vi "Find Device by Multicolumn Listbox Value.vi"(3 "error in (no error)":errorcluster, 4 "Multicolumn Listbox":refnum<vi>, 5 "ACNET Devices":refnum<class "ACNET Devices.lvclass">) -> (0 "error out":errorcluster, 1 "Found?":bool, 2 "ACNET Device Cluster":T1)   [LabVIEW 2013, in "ACNET Monitor.lvlib"]
uses:
  ACNET Monitor.lvlib
  ACNET Devices.lvclass
  ACNET Device.lvclass
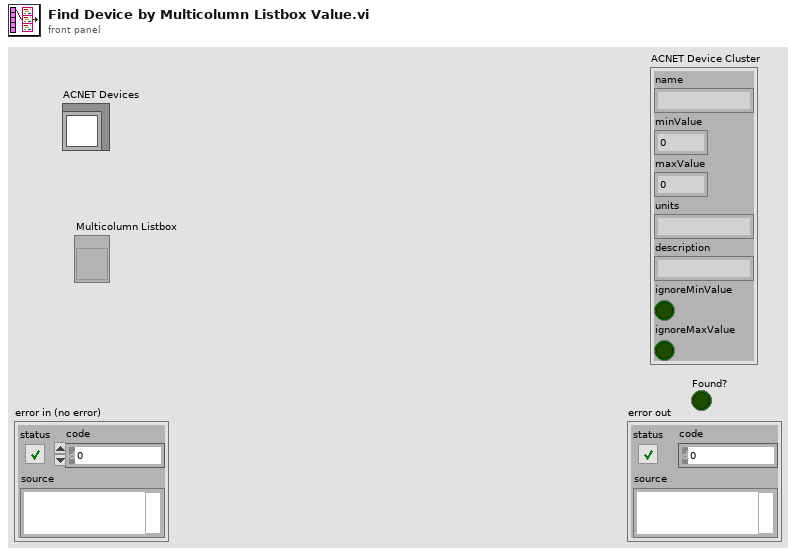
[diagram p1: front panel]
types:
  T1 = cluster{"name":string, "minValue":dbl, "maxValue":dbl, "units":string, "description":string, "ignoreMinValue":bool, "ignoreMaxValue":bool}
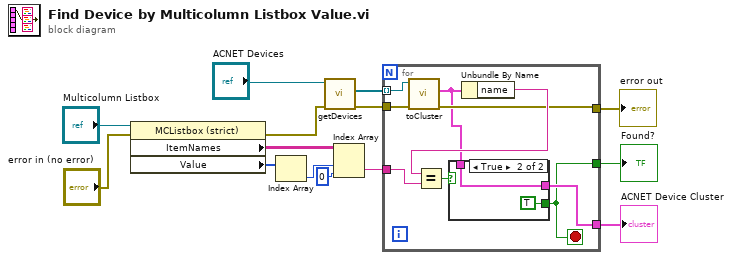
[diagram p0: block diagram]
diagram:
  n1 = property on="Property Node" class="MCListbox (strict)"(reference="Multicolumn Listbox", error in="error in (no error)") -> (error out=w10:errorcluster, "ItemNames"=w13:string[][], "Value"=w7:i32[])  [unwired: 1 out]
  n2 = Index Array(array=w7) -> (element=w14:i32)  [unwired: 1 in]
  n3 = call-dynamic "getDevices.vi"("error in (no error)"=w10, "ACNET Devices in"="ACNET Devices") -> ("error out"=w12:errorcluster, "Devices"=w11:refnum<class "ACNET Device.lvclass">[])  [unwired: 7 in, 1 out]
  n4 = Index Array(array=w13, index (row)=w14, index (col)=0 ("disabled index (col)")) -> (element=w1:string)
  n5 = for {
    tunnel: w11 -> [w23] mode=indexing
    tunnel: w12 -> [w22]
    tunnel: w1 -> [w20]
    tunnel: [w18] -> w5
    tunnel: [w16] -> w3
    tunnel: [w15] -> w4
    stop <- w15 stop-if-true
    n6 = call-dynamic "toCluster.vi"("error in (no error)"=w22, "ACNET Device in"=w23) -> ("error out"=w18:errorcluster, "ACNET Device Cluster"=w17:T1)  [unwired: 7 in, 1 out]
    n7 = Unbundle By Name(w17) -> ("name"=w21:string)
    n8 = Equal?(x=w21, y=w20) -> (x = y?=w19:bool)
    n9 = case shown="True" w19 {
      tunnel: [_ TRUE] -> w15
      tunnel: w17 -> [_ w24]
      tunnel: [_ w24] -> w16
      frame False {
      }
      frame True {
      }
    }
  }
  "error out" <- w5
  "Found?" <- w4
  "ACNET Device Cluster" <- w3
